vi "Upload Package.vi"   [LabVIEW 2021]
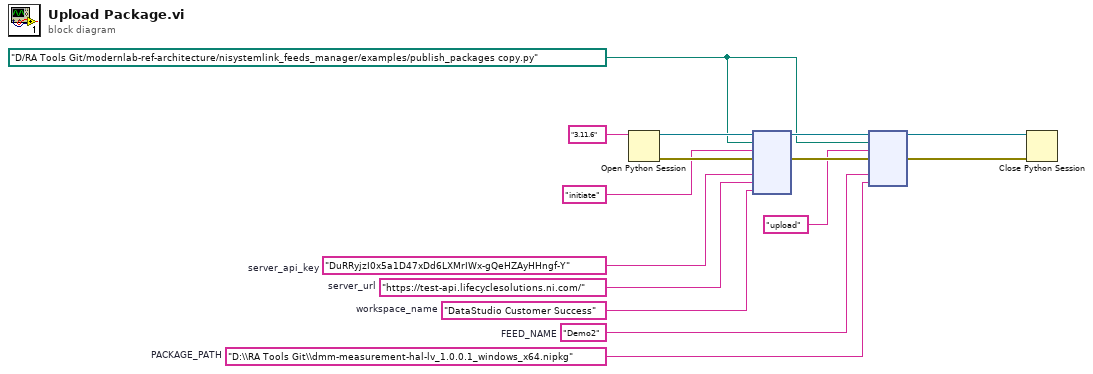
[diagram p0: block diagram]
diagram:
  w1 = "D:\\RA Tools Git\\dmm-measurement-hal-lv_1.0.0.1_windows_x64.nipkg"  # PACKAGE_PATH
  w2 = "Demo2"  # FEED_NAME
  w9 = "DataStudio Customer Success"  # workspace_name
  w10 = "https://test-api.lifecyclesolutions.ni.com/"  # server_url
  w11 = "DuRRyjzI0x5a1D47xDd6LXMrIWx-gQeHZAyHHngf-Y"  # server_api_key
  w3 = path "D:/RA Tools Git/modernlab-ref-architecture/nisystemlink_feeds_manager/examples/publish_packages copy.py" ("module path")
  n1 = Open Python Session(python version="3.11.6" ("Python version")) -> (session out=w14:refnum<k35>, error out=w13:errorcluster)  [unwired: 2 in]
  n2 = node(w14, w3, "initiate" ("function name"), w13, w11, w10, w9) -> (w8:refnum<k35>, w6:errorcluster)  [unwired: 5 in, 2 out]
  n3 = node(w8, w3, "upload" ("function name"), w6, w2, w1) -> (w7:refnum<k35>, w5:errorcluster)  [unwired: 4 in, 2 out]
  n4 = Close Python Session(session in=w7, error in=w5) -> ()  [unwired: 1 out]
